vi "SLAM_main.vi"(8 "measurements":dbl[][](array[numeric]), 9 "dX":dbl[](array[numeric]), 10 "P":dbl[][](array[numeric]), 11 "X":dbl[](array[numeric])) -> (0 "measuredLandmarks":dbl[][](array[numeric]), 1 "Xodometry":dbl[](array[numeric]), 2 "Pout":dbl[][](array[numeric]), 3 "Xout":dbl[](array[numeric]))   [LabVIEW 2009, in "LV_SLAM.lvlib"]
uses:
  LV_SLAM.lvlib
  <vilib>/Analysis/Matrix/Numeric/Conversions/Array To Matrix - RA2.vi
  <vilib>/Analysis/Matrix/NI_Matrix.lvlib
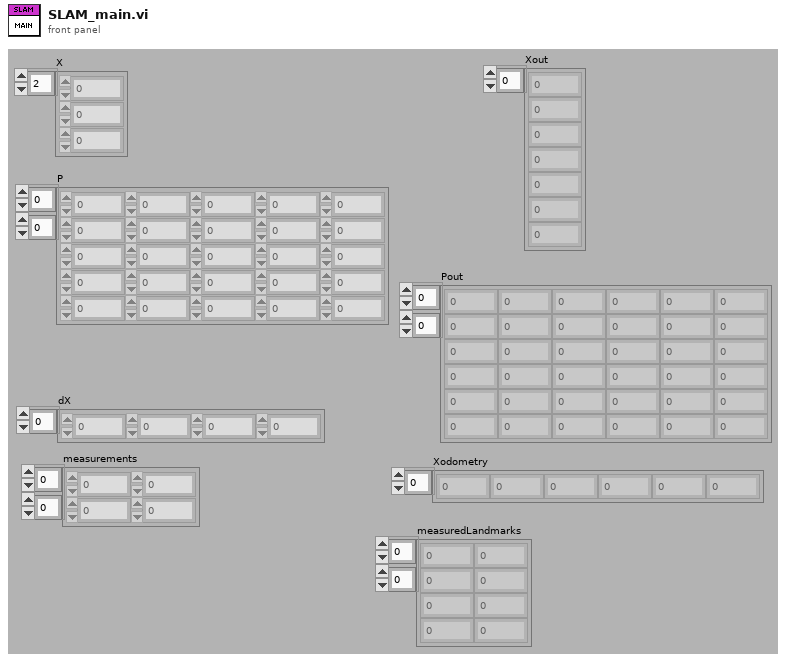
[diagram p1: front panel]
types:
  T1 = typedef "NI_Matrix.lvlib/RealMatrix.ctl" = dbl[][]
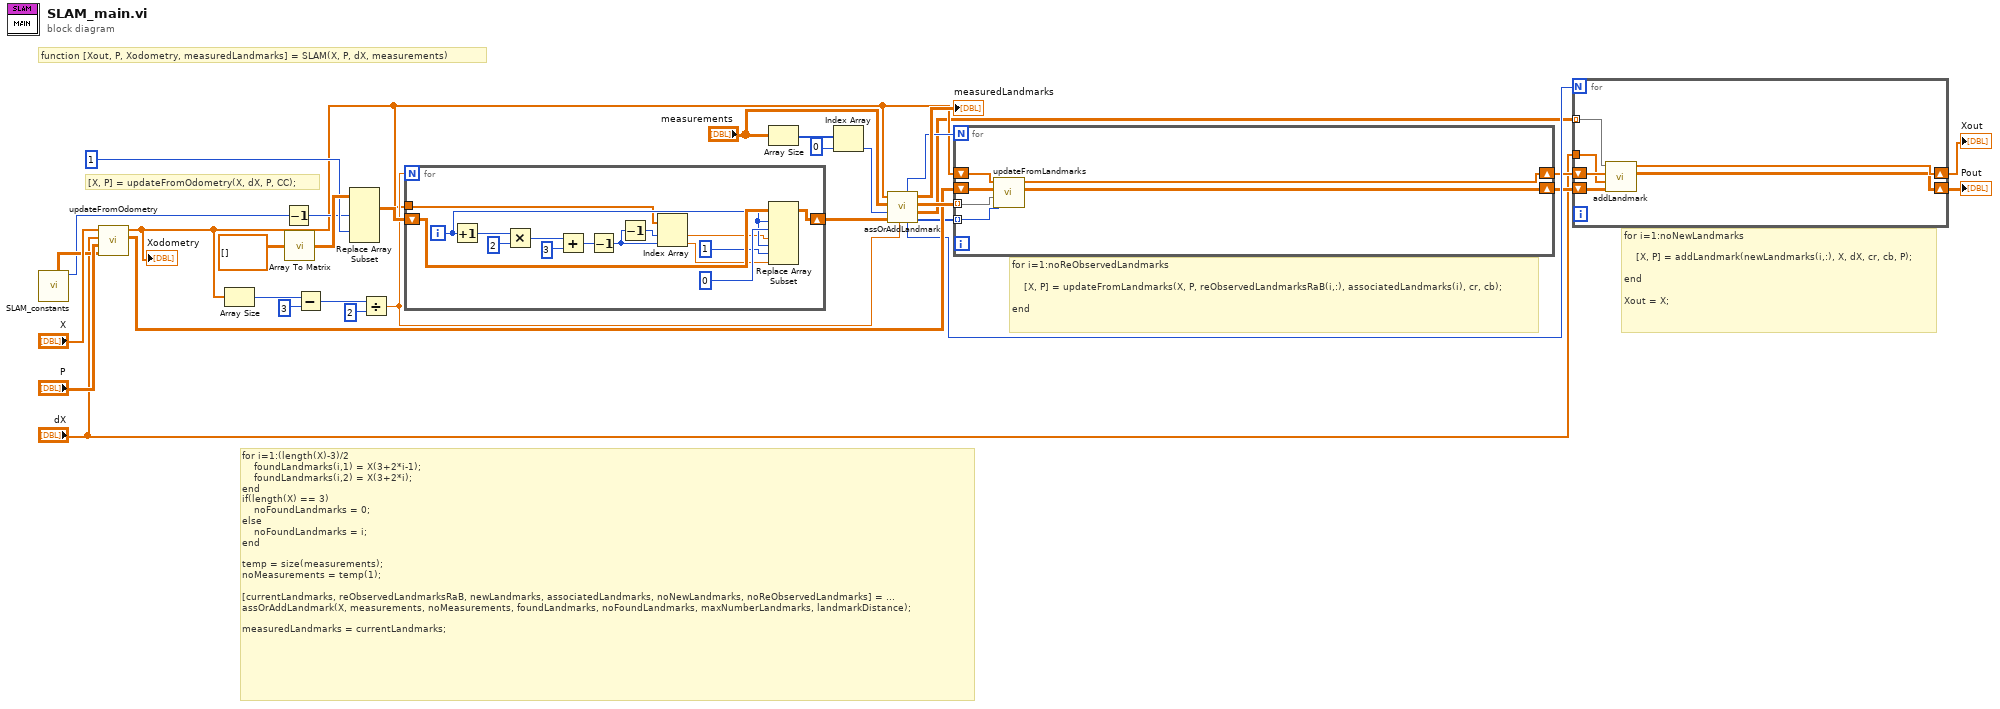
[diagram p0: block diagram]
diagram:
  # "function [Xout, P, Xodometry, measuredLandmarks] = SLAM(X, P, dX, measurements)"
  # "[X, P] = updateFromOdometry(X, dX, P, CC);"
  # "for i=1:noNewLandmarks\n\n    [X, P] = addLandmark(newLandmarks(i,:), X, dX, cr, cb, P);\n\nend\n\nXout = X;"
  # "for i=1:noReObservedLandmarks\n\n    [X, P] = updateFromLandmarks(X, P, reObservedLandmarksRaB(i,:), associatedLandmarks(i), cr, cb);\n\nend"
  # "for i=1:(length(X)-3)/2\n    foundLandmarks(i,1) = X(3+2*i-1);\n    foundLandmarks(i,2) = X(3+2*i);\nend\nif(length(X) == 3)\n    noFoundLandmarks = 0;\nelse\n    noFoundLandmarks = i;\nend\n\ntemp = size(measurements);\nnoMeasurements = temp(1);\n\n[currentLandmarks, reObservedLandmarksRaB, newLandmarks, associatedLandmarks, noNewLandmarks, noReObservedLandmarks] = ...\nassOrAddLandmark(X, measurements, noMeasurements, foundLandmarks, noFoundLandmarks, maxNumberLandmarks, landmarkDistance);\n\nmeasuredLandmarks = currentLandmarks;"
  n1 = call "SLAM_constants.vi"() -> ("maxNumberLandmarks"=w25:i32, "CC"=w26:T1)  [unwired: 7 in, 3 out]
  n2 = call "updateFromOdometry.vi"("CC"=w26, "P"="P", "dX"="dX", "X"="X") -> ("P out"=w9:dbl[][], "X out"=w10:dbl[])  [unwired: 6 in]
  "Xodometry" <- w10
  n3 = Array Size(array=w10) -> (size(s)=w24:i32)
  n4 = Decrement(x=w25) -> (x-1=w27:i32)
  n5 = call-poly <vilib>:"Array To Matrix.vi"("Real 2D Array"=dbl[][] [] ("foundLandmarks")) -> ("Real Matrix"=w30:T1)
  n6 = Subtract(x=w24, y=3) -> (x-y=w22:i32)
  n7 = Replace Array Subset(array=w30, index (dim 1)=w27, index (dim 3)=1 ("column N")) -> (w20:T1)  [unwired: 3 in]
  n8 = Divide(x=w22, y=2) -> (x/y=w14:dbl)
  n9 = for {
    N: w14 -> [_]
    tunnel: w10 -> [w38]
    shift-right: [w44] -> w15
    shift-left: w20 -> [w47]
    i -> [w40]
    n10 = Increment(x=w40) -> (x+1=w33:i32)
    n11 = Multiply(x=w33, y=2) -> (x*y=w42:i32)
    n12 = Add(x=w42, y=3) -> (x+y=w39:i32)
    n13 = Decrement(x=w39) -> (x-1=w37:i32)
    n14 = Decrement(x=w37) -> (x-1=w36:i32)
    n15 = Index Array(array=w38, index #1=w36, index #2=w37) -> (element #1=w35:dbl, element #2=w34:dbl)
    n16 = Replace Array Subset(array=w47, new element #1=w35, index (row) #1=w40, index (col) #1=0 ("index"), new element #2=w34, index (row) #2=w40, index (col) #2=1 ("index")) -> (w44:T1)
  }
  n17 = Array Size(array="measurements") -> (size(s)=w19:i32[])
  n18 = Index Array(array=w19, index=0) -> (element=w17:i32)
  n19 = call "assOrAddLandmark.vi"("noFoundLandmarks"=w14, "foundLandmarks"=w15, "noMeasurements"=w17, "measurements"="measurements", "X"=w10) -> ("associatedLandmarks"=w8:i32[], "newLandmarks"=w6:dbl[][], "reObservedLandmarksRaB"=w11:dbl[][], "currentLandmarks"=→"measuredLandmarks":dbl[][], "noNewLandmarks"=w7:i32, "noReObservedLandmarks"=w12:i32)  [unwired: 1 in]
  n20 = for {
    N: w12 -> [_]
    tunnel: w11 -> [w51] mode=indexing
    shift-right: [w48] -> w4
    shift-left: w9 -> [w52]
    shift-right: [w49] -> w5
    shift-left: w10 -> [w53]
    tunnel: w8 -> [w50] mode=indexing
    n21 = call "updateFromLandmarks.vi"("landmarkNumber"=w50, "measurement"=w51, "P"=w52, "X"=w53) -> ("P out"=w48:dbl[][], "X out"=w49:dbl[])  [unwired: 6 in]
  }
  n22 = for {
    N: w7 -> [_]
    tunnel: w6 -> [w59] mode=indexing
    shift-right: [w55] -> w2
    shift-left: w5 -> [w58]
    shift-right: [w54] -> w1
    shift-left: w4 -> [w56]
    tunnel: "dX" -> [w57]
    n23 = call "addLandmark.vi"("P"=w56, "dX"=w57, "X"=w58, "newLandmark"=w59) -> ("P out"=w54:dbl[][], "X out"=w55:dbl[])  [unwired: 6 in]
  }
  "Pout" <- w1
  "Xout" <- w2
